vi "FastMap - Safe Move.vi"(8 "Action Order":cluster{"Action":T2, "Direction":T1}[](array[cluster]), 9 "Column":i32, 10 "Row":i32, 11 "fast map in":refnum<data-value>) -> (1 "Selected Direction":T1, 2 "Selected Action":T2, 3 "fast map out":refnum<data-value>)   [LabVIEW 2015, in "DS Square.lvlib"]
uses:
  DS Square.lvlib
  Common/Position.ctl
  Common/Common.lvlib
  Type Defs/Direction Enum.ctl
  Type Defs/SB Type Defs.lvlib
  Type Defs/Action Enum.ctl
  Square State Fast.ctl
  Fast Map.ctl
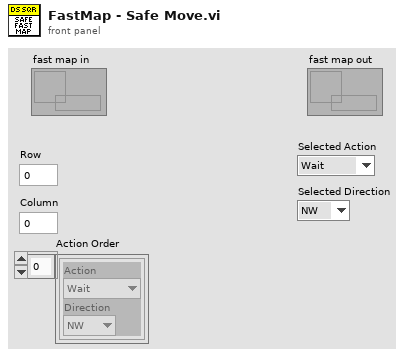
[diagram p1: front panel]
types:
  T1 = typedef "SB Type Defs.lvlib/Direction Enum.ctl" = enum16{"NW", "N", "NE", "E", "SE", "S", "SW", "W"}
  T2 = typedef "SB Type Defs.lvlib/Action Enum.ctl" = enum16{"Wait", "Move", "Attack", "Replicate"}
  T3 = typedef "Common.lvlib/Position.ctl" = cluster{"Column":i32, "Row":i32}
  T4 = typedef "DS Square.lvlib/Square State Fast.ctl" = enum8{"Unknown", "Empty", "Occupied - Active", "Occupied - Cool Down", "Attacked", "Enemy", "Enemy Wall"}
  T5 = typedef "DS Square.lvlib/Fast Map.ctl" = cluster{"state":T4[][], "updated":i32[][]}
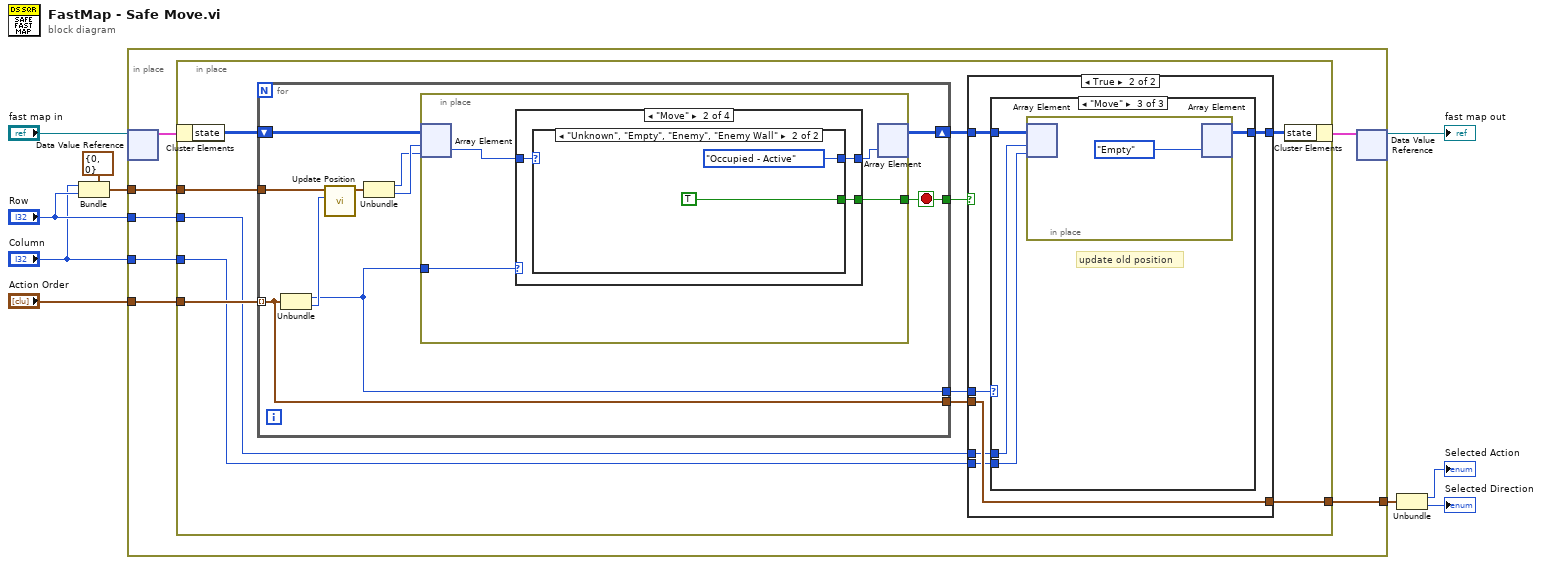
[diagram p0: block diagram]
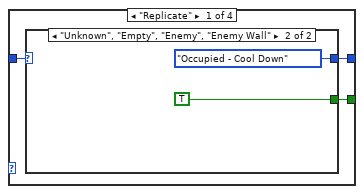
[diagram p2: hidden frame]
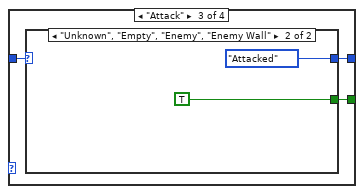
[diagram p5: hidden frame]
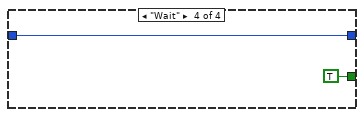
[diagram p7: hidden frame]
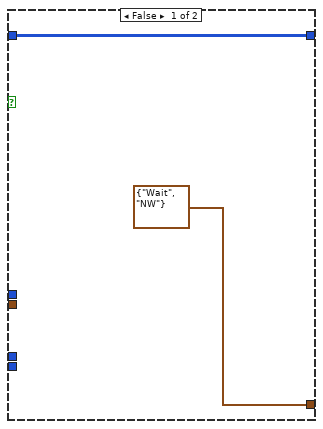
[diagram p8: hidden frame]
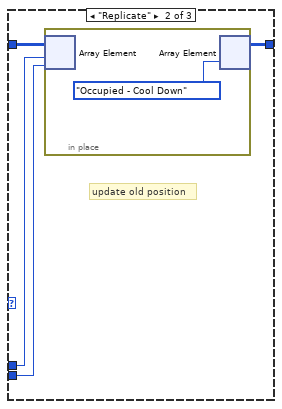
[diagram p10: hidden frame]
diagram:
  n1 = Bundle(cluster=T3 {"Column"=0, "Row"=0} ("Position in"), "Column"="Column", "Row"="Row") -> (w6:T3)
  n2 = in-place {
    in-place-border: "Action Order" -> [w15]
    in-place-border: w6 -> [w14]
    in-place-border: [w13] -> w5
    in-place-border: "Row" -> [w12]
    in-place-border: "Column" -> [w11]
    n3 = in-place-dvr #1("fast map in") -> (w17:T5)  [unwired: 1 out]
    n4 = in-place {
      in-place-border: w15 -> [w27]
      in-place-border: w14 -> [w26]
      in-place-border: [w23] -> w13
      in-place-border: w12 -> [w21]
      in-place-border: w11 -> [w20]
      n5 = in-place-cluster #2(w17) -> ("state"=w28:T4[][])
      n6 = for {
        shift-right: [w35] -> w25
        shift-left: w28 -> [w37]
        tunnel: w27 -> [w32] mode=indexing
        tunnel: [w34] -> w19
        tunnel: [w33] -> w22
        tunnel: [w32] -> w24
        tunnel: w26 -> [w29]
        stop <- w33 stop-if-true
        n7 = Unbundle(w32) -> ("Action"=w34:T2, "Direction"=w36:T1)
        n8 = call "Update Position.vi"("Direction"=w36, "Position in"=w29) -> ("Position out"=w38:T3)  [unwired: 9 in]
        n9 = Unbundle(w38) -> ("Column"=w30:i32, "Row"=w31:i32)
        n10 = in-place {
          in-place-border: [w42] -> w33
          in-place-border: w34 -> [w41]
          n11 = in-place-array #3(w37, w31, w30) -> (w40:T4)
          n12 = case shown="\"Move\"" w41 {
            tunnel: w40 -> [w45 w51 w57 w62]
            tunnel: [w44 w50 w56 w62] -> w39
            tunnel: [w43 w49 w55 TRUE] -> w42
            frame "Replicate" {
              n13 = case shown="\"Unknown\", \"Empty\", \"Enemy\", \"Enemy Wall\"" w45 {
                selector: w45 -> [w46 _]
                tunnel: [w46 Square_State_Fast."Occupied - Cool Down" ("square state")] -> w44
                tunnel: [_ TRUE] -> w43
                frame "Occupied - Active".."Attacked" {
                }
                frame "Unknown", "Empty", "Enemy", "Enemy Wall" {
                }
              }
            }
            frame "Move" {
              n14 = case shown="\"Unknown\", \"Empty\", \"Enemy\", \"Enemy Wall\"" w51 {
                selector: w51 -> [w52 _]
                tunnel: [w52 Square_State_Fast."Occupied - Active" ("square state")] -> w50
                tunnel: [_ TRUE] -> w49
                frame "Occupied - Active".."Attacked" {
                }
                frame "Unknown", "Empty", "Enemy", "Enemy Wall" {
                }
              }
            }
            frame "Attack" {
              n15 = case shown="\"Unknown\", \"Empty\", \"Enemy\", \"Enemy Wall\"" w57 {
                selector: w57 -> [w58 _]
                tunnel: [w58 Square_State_Fast."Attacked" ("square state")] -> w56
                tunnel: [_ TRUE] -> w55
                frame "Occupied - Active".."Attacked" {
                }
                frame "Unknown", "Empty", "Enemy", "Enemy Wall" {
                }
              }
            }
            frame "Wait" {
            }
          }
          n16 = in-place-array #3(w39) -> (w35:T4[][])  [unwired: 2 out]
        }
      }
      n17 = case shown="True" w22 {
        tunnel: w25 -> [w64 w70]
        tunnel: w19 -> [_ w69]
        tunnel: [w64 w68] -> w18
        tunnel: w24 -> [_ w67]
        tunnel: [cluster{"Action":T2, "Direction":T1} {"Action"=enum."Wait", "Direction"=enum."NW"} w67] -> w23
        tunnel: w21 -> [_ w66]
        tunnel: w20 -> [_ w65]
        frame False {
        }
        frame True {
          n18 = case shown="\"Move\"" w69 {
            tunnel: w70 -> [w71 w75 w80]
            tunnel: [w71 w74 w79] -> w68
            tunnel: w66 -> [_ w73 w77]
            tunnel: w65 -> [_ w72 w78]
            frame Default {
            }
            frame "Replicate" {
              # "update old position"
              n19 = in-place {
                n20 = in-place-array #4(w75, w73, w72) -> ()  [unwired: 1 out]
                n21 = in-place-array #4(Square_State_Fast."Occupied - Cool Down" ("square state")) -> (w74:T4[][])  [unwired: 2 out]
              }
            }
            frame "Move" {
              # "update old position"
              n22 = in-place {
                n23 = in-place-array #5(w80, w77, w78) -> ()  [unwired: 1 out]
                n24 = in-place-array #5(Square_State_Fast."Empty" ("square state")) -> (w79:T4[][])  [unwired: 2 out]
              }
            }
          }
        }
      }
      n25 = in-place-cluster #2("state"=w18) -> (w16:T5)
    }
    n26 = in-place-dvr #1(w16) -> (→"fast map out":refnum<data-value>)  [unwired: 1 out]
  }
  n27 = Unbundle(w5) -> ("Action"=→"Selected Action":T2, "Direction"=→"Selected Direction":T1)
